vi "_PC_Pub_FM signalToTDMS.vi"(8 "error in (no error)":errorcluster, 11 "SignalData":waveform(sgl)) -> (0 "error out":errorcluster, 3 "dataParam":T1, 5 "attrType":i16[](array[numeric]))   [LabVIEW 2018, in "FM.lvclass"]
uses:
  FM.lvclass
  Overload/Experiment Condition/_PC_Pub_ExpCondiValue_SignalRemarks.vi
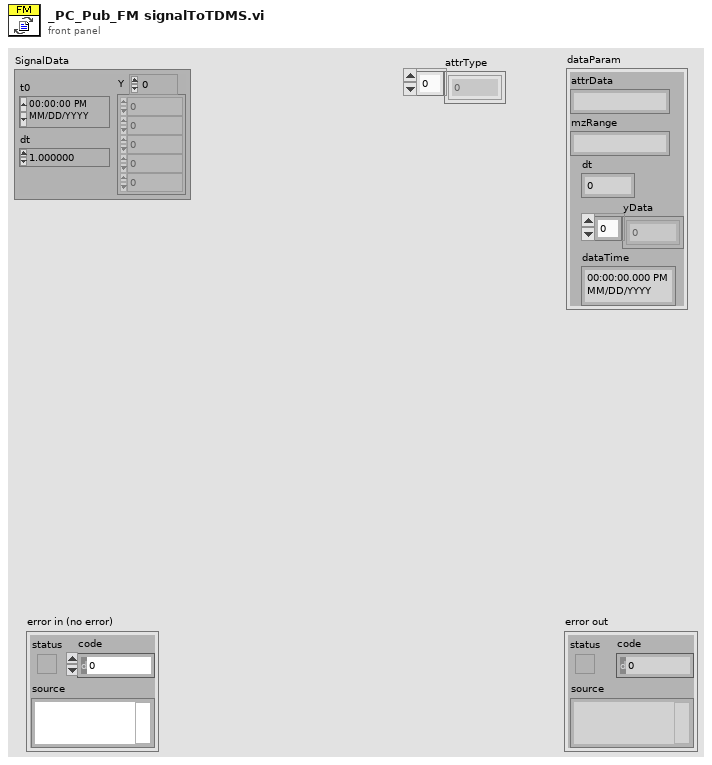
[diagram p1: front panel]
types:
  T1 = cluster{"attrData":string, "mzRange":string, "dt":dbl, "yData":sgl[], "dataTime":timestamp}
  T2 = cluster{"attrData":string, "mzRange":string, "dt":dbl, "yData":sgl[], "t0":timestamp}
  T3 = cluster{"InfoID":u64, "SignalInfo":cluster{"Label":string, "dt":dbl, "Length":u32, "RefVolt":dbl, "mzTable":cluster{"t":dbl[], "mz":dbl[], "beta":dbl[]}}[]}
  T4 = cluster{"Label":string, "dt":dbl, "Length":u32, "RefVolt":dbl, "mzTable":cluster{"t":dbl[], "mz":dbl[], "beta":dbl[]}}[]
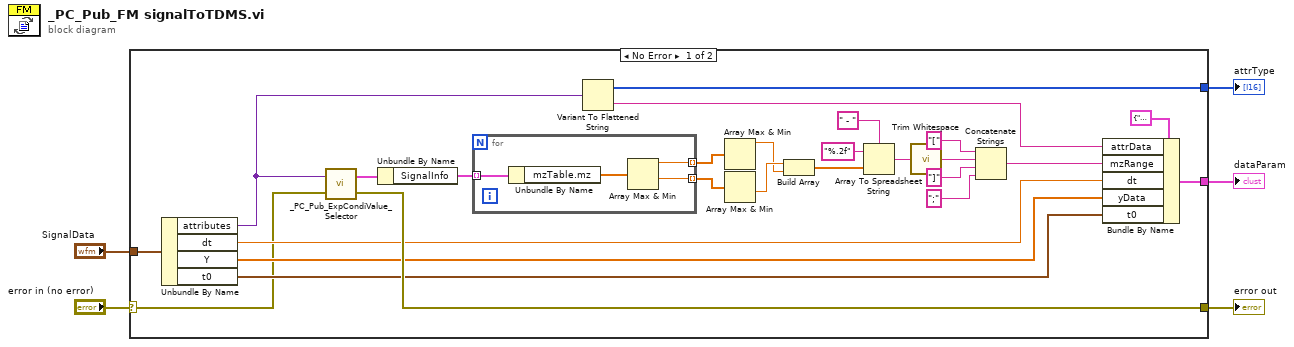
[diagram p0: block diagram]
diagram:
  n1 = case shown="No Error" "error in (no error)" {
    selector: "error in (no error)" -> [w7 w36]
    tunnel: [w30 w36] -> w4
    tunnel: "SignalData" -> [w31 _]
    tunnel: [w17 _] -> w2
    tunnel: [w11 _] -> w1
    frame No Error {
      n2 = Unbundle By Name(w31) -> ("attributes"=w6:variant, "dt"=w13:dbl, "Y"=w12:sgl[], "t0"=w10:timestamp)
      n3 = call-poly "_PC_Pub_ExpCondiValue_Selector.vi"("error in (no error)"=w7, "expCondiVariant"=w6) -> ("error out"=w30:errorcluster, "SignalRemarks"=w29:T3)
      n4 = Unbundle By Name(w29) -> ("SignalInfo"=w28:T4)
      n5 = for {
        tunnel: w28 -> [w35] mode=indexing
        tunnel: [w33] -> w26 mode=indexing
        tunnel: [w32] -> w27 mode=indexing
        n6 = Unbundle By Name(w35) -> ("mzTable.mz"=w34:dbl[])
        n7 = Array Max & Min(array=w34) -> (max value=w32:dbl, min value=w33:dbl)  [unwired: 2 out]
      }
      n8 = Variant To Flattened String(Variant=w6) -> (data string=w14:string, 1:w17:i16[])
      n9 = Array Max & Min(array=w27) -> (max value=w18:dbl)  [unwired: 3 out]
      n10 = Array Max & Min(array=w26) -> (min value=w19:dbl)  [unwired: 3 out]
      n11 = Build Array(w19, w18) -> (w23:dbl[])
      n12 = Array To Spreadsheet String(delimiter (Tab)=" - ", array=w23, 3:"%.2f" ("format string")) -> (spreadsheet string=w9:string)
      n13 = call <vilib>:"Trim Whitespace.vi"("string"=w9) -> ("trimmed string"=w8:string)  [unwired: 1 in]
      n14 = Concatenate Strings("[" ("string"), w8, "]" ("string"), ";" ("string")) -> (w15:string)
      n15 = Bundle By Name(cluster=T2 {"attrData"="", "mzRange"="", "dt"=0.0, "yData"=[], "t0"=timestamp(0 s since 1904-01-01)}, "attrData"=w14, "mzRange"=w15, "dt"=w13, "yData"=w12, "t0"=w10) -> (w11:T2)
    }
    frame Error {
    }
  }
  "error out" <- w4
  "attrType" <- w2
  "dataParam" <- w1
